vi "MergeTool - Cambridge.vi"(8 "VI Reference":refnum<vi>, 10 "Display References":refnum<vi>[](array[refnum])) -> ()   [LabVIEW 2014]
uses:
  <vilib>/Utility/cursorutil.llb/Set Cursor (Icon Pict).vi
panel:
  in  "Save":bool
  in  "Reset Zoom":bool
  in  "Zoom In":bool
  in  "Pick Blue":bool
  in  "Pick Green":bool
  in  "Pick Red":bool
  in  "Clear All":bool
  out "Merge Image":picture
  in  "Exit":bool
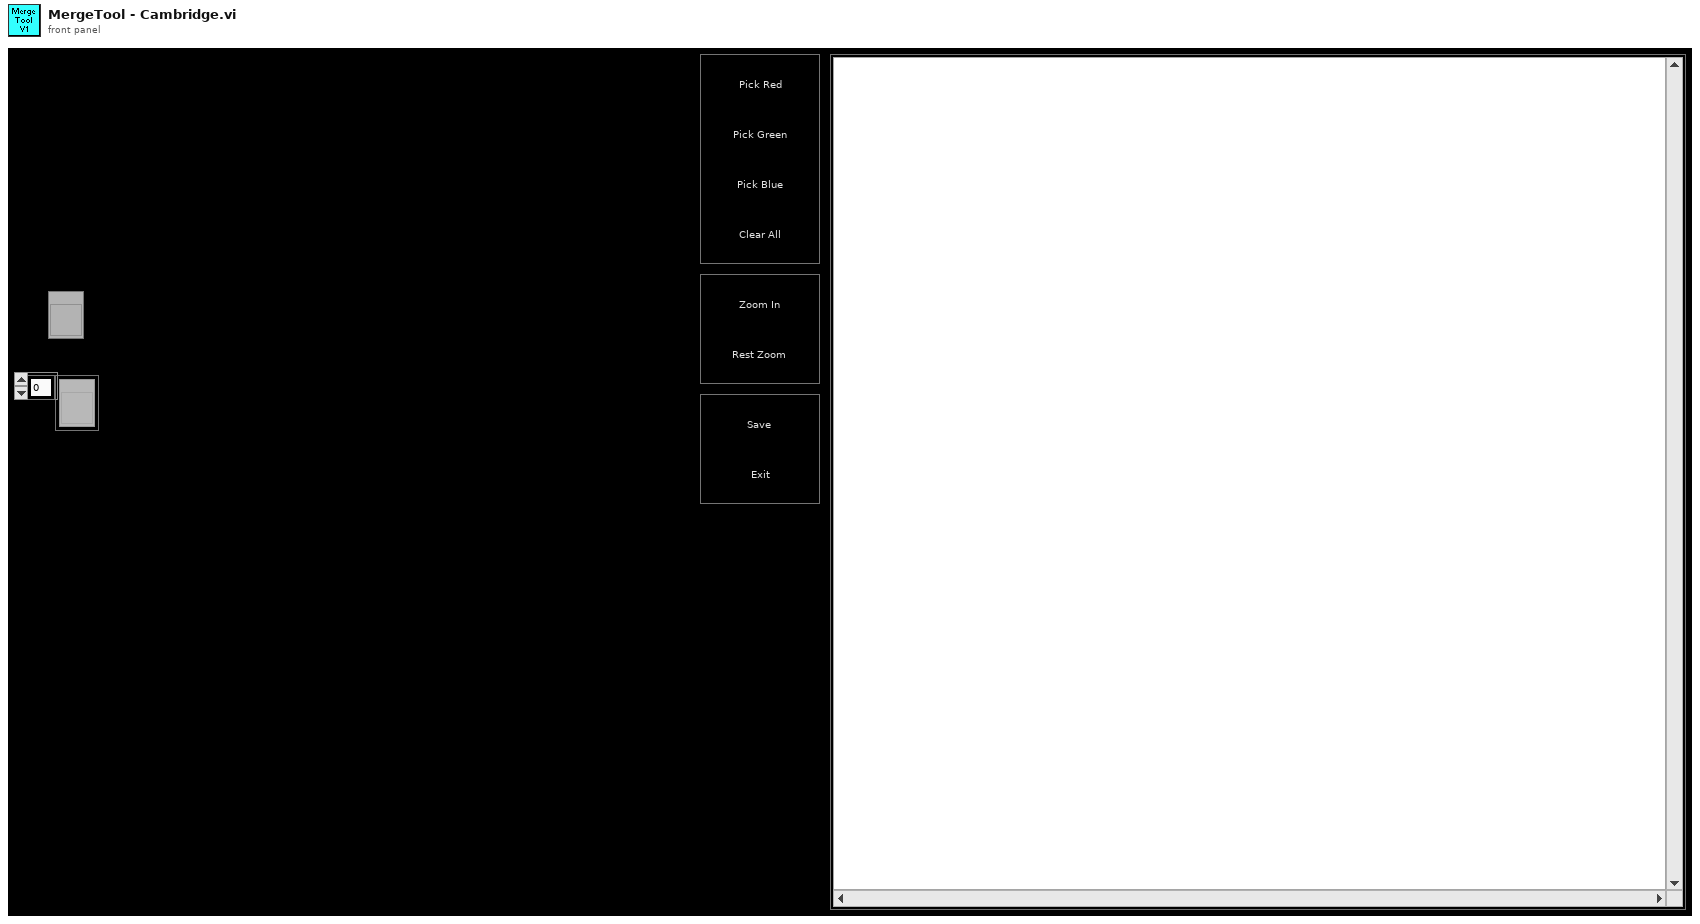
[diagram p1: front panel]
types:
  T1 = typedef "LVBoundsTypeDef.ctl" = cluster{"Width":u32, "Height":u32}
  T2 = typedef "imagedata.ctl" = cluster{"image type":i32, "image depth":i32, "image":u8[], "mask":u8[], "colors":u32[], "Rectangle":cluster{"left":i16, "top":i16, "right":i16, "bottom":i16}}
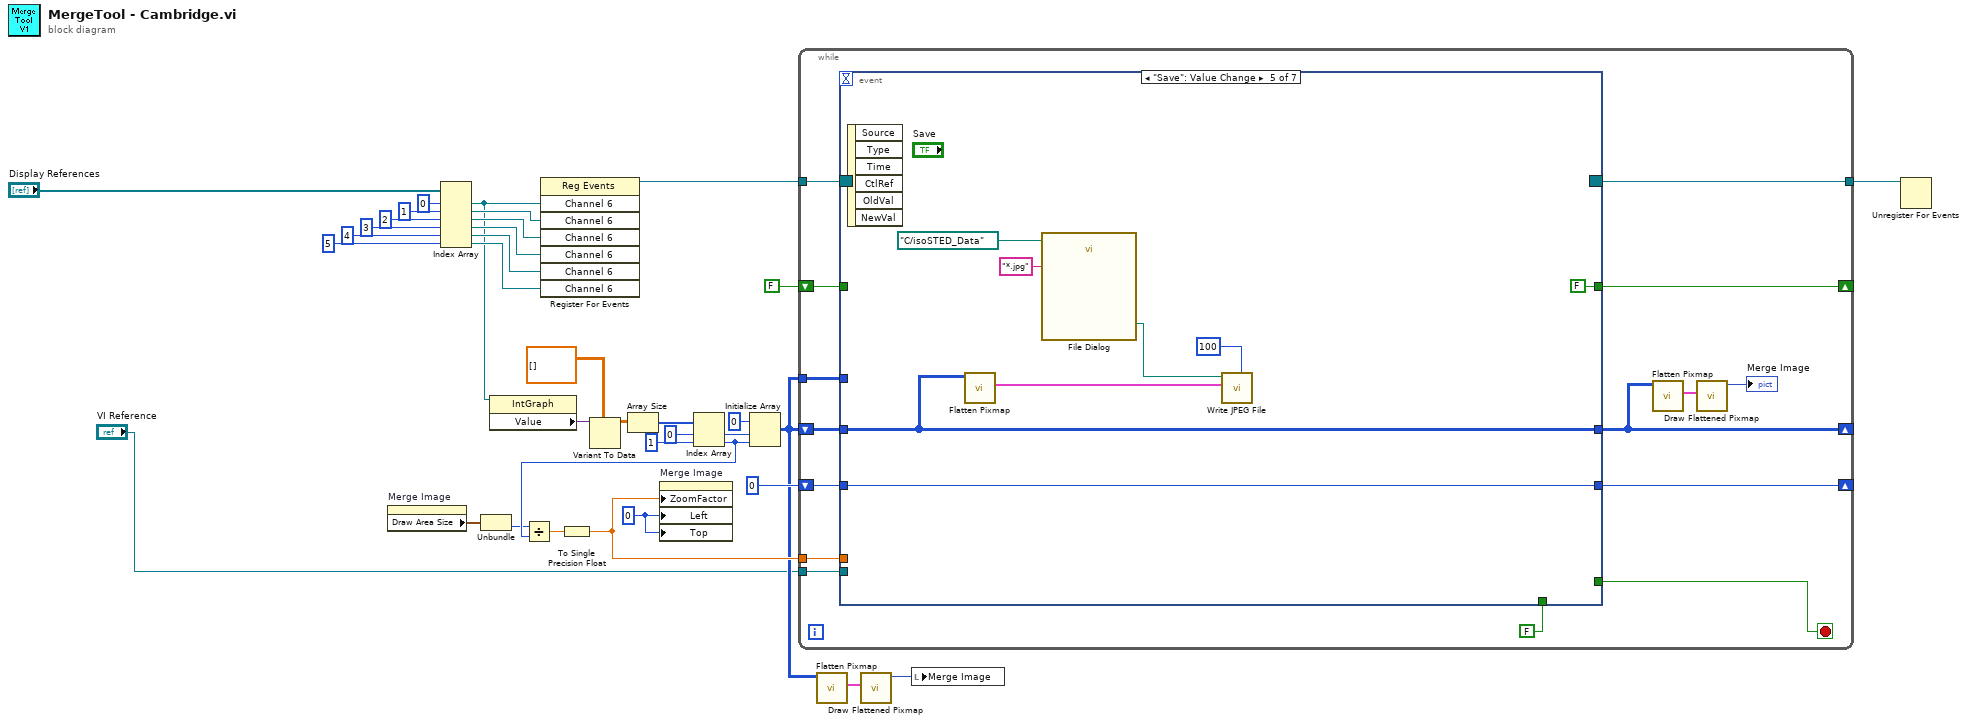
[diagram p0: block diagram]
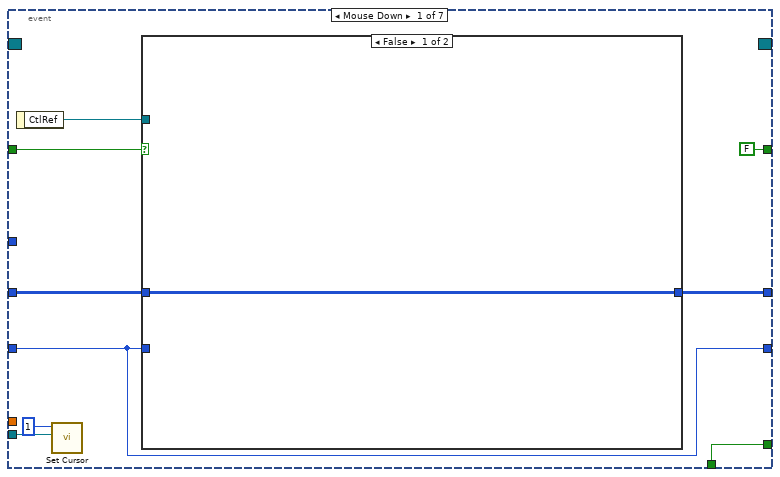
[diagram p2: hidden frame]
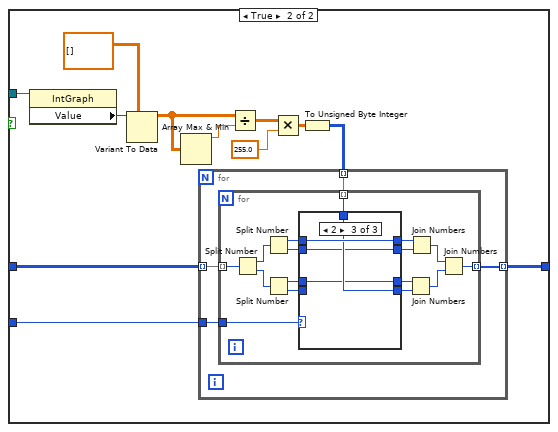
[diagram p3: hidden frame]
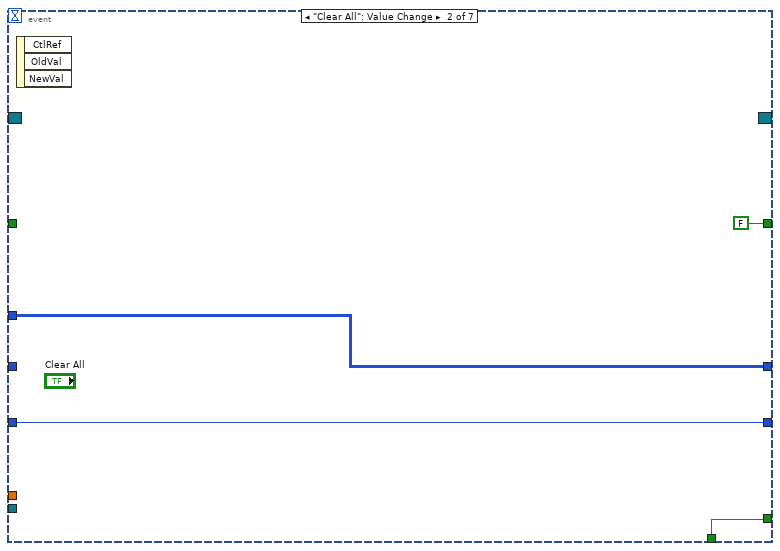
[diagram p6: hidden frame]
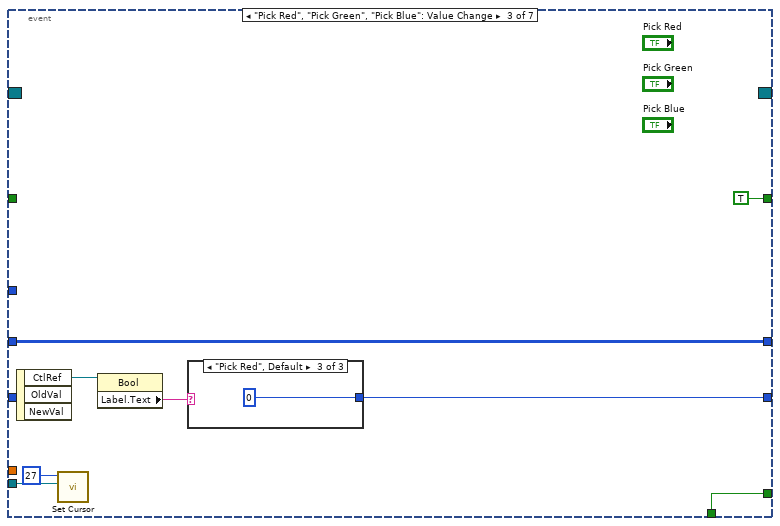
[diagram p7: hidden frame]
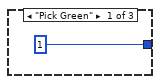
[diagram p8: hidden frame]
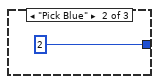
[diagram p9: hidden frame]
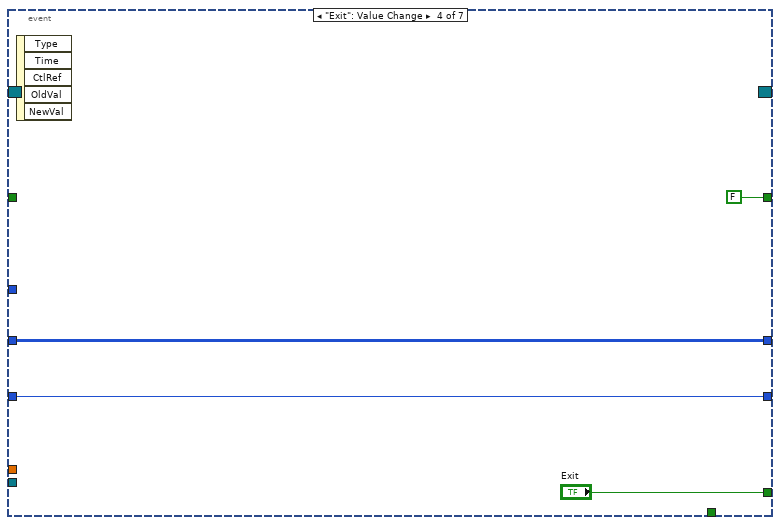
[diagram p10: hidden frame]
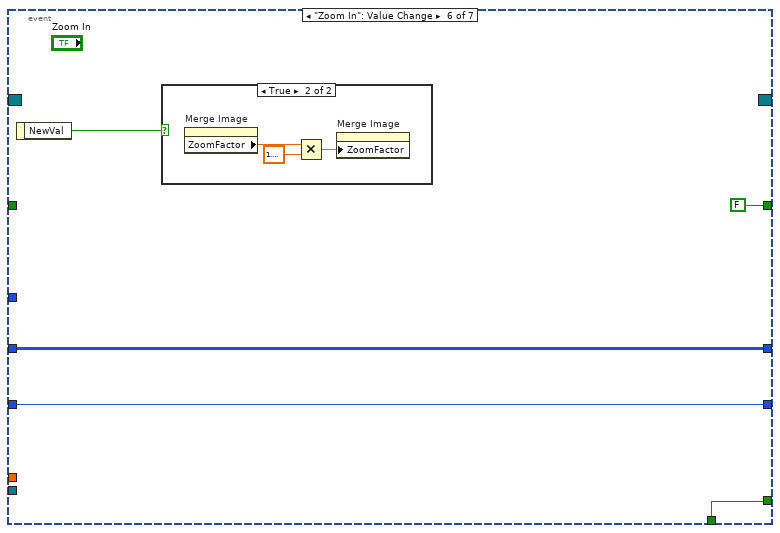
[diagram p11: hidden frame]
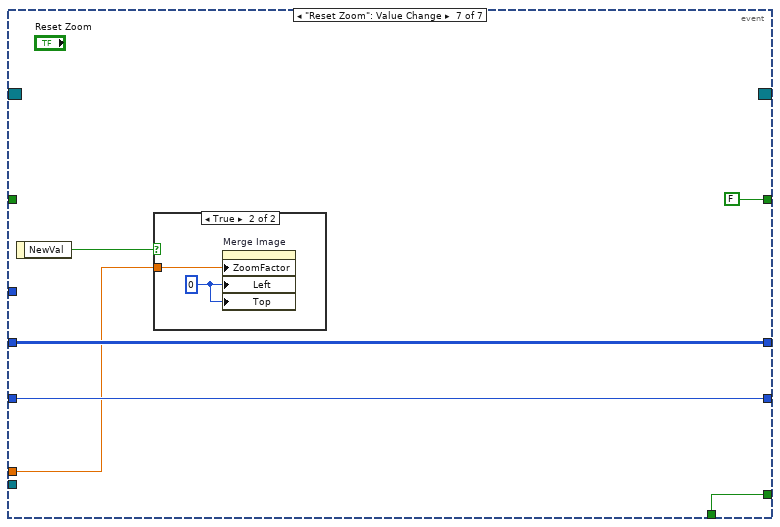
[diagram p13: hidden frame]
diagram:
  w7 = i16 0 ("Origin:Left")
  n1 = property on="Merge Image" class="Pict"() -> ("Draw Area Size"=w12:T1)  [unwired: 2 in, 2 out]
  n2 = Index Array(array="Display References", index #1=0 ("index"), index #2=1 ("index"), index #3=2 ("index"), index #4=3 ("index"), index #5=4 ("index"), index #6=5 ("index")) -> (element #1=w22:refnum<vi>, element #2=w25:refnum<vi>, element #3=w26:refnum<vi>, element #4=w27:refnum<vi>, element #5=w28:refnum<vi>, element #6=w29:refnum<vi>)
  n3 = Unbundle(w12) -> ("Height"=w11:u32)  [unwired: 1 out]
  n4 = property class="IntGraph"(reference=w22) -> ("Value"=w21:variant)  [unwired: 1 in, 2 out]
  n5 = register-events(w22, w25, w26, w27, w28, w29) -> (reference out=w24:refnum<event-registration>)  [unwired: 2 in, 1 out]
  n6 = Variant To Data(type=sgl[][] [], Variant=w21) -> (data=w19:sgl[][])  [unwired: 1 in, 1 out]
  n7 = Array Size(array=w19) -> (size(s)=w18:i32[])
  n8 = Index Array(array=w18, index #1=0 ("index"), index #2=1 ("index")) -> (element #1=w15:i32, element #2=w13:i32)
  n9 = Divide(x=w11, y=w13) -> (x/y=w9:dbl)
  n10 = To Single Precision Float(number=w9) -> (single precision float=w8:sgl)
  n11 = property on="Merge Image" class="Pict"("ZoomFactor"=w8, "Left"=w7, "Top"=w7) -> ()  [unwired: 2 in, 2 out]
  n12 = Initialize Array(u32 0 ("element"), w15, w13) -> (w4:u32[][])
  n13 = while {
    tunnel: w24 -> [w48]
    tunnel: [w47] -> w23
    shift-right: [w42] -> _
    shift-left: w4 -> [w46]
    tunnel: w4 -> [w45]
    tunnel: "VI Reference" -> [w41]
    shift-right: [w40] -> _
    shift-left: u8 0 -> [w39]
    tunnel: w8 -> [w38]
    shift-right: [w37] -> _
    shift-left: FALSE -> [w36]
    stop <- w50 stop-if-true
    n14 = event shown="[4] \"Save\": Value Change" {
      selector: w48 -> [_ _ _ _ _ _ _]
      dyn-events: [_ _ _ _ _ _ _] -> w47
      timeout: _ -> [_ _ _ _ _ _ _]
      tunnel: [w58 w107 w116 "Exit" _ w136 w143] -> w50
      tunnel: FALSE -> [w58 w107 w116 _ _ w136 w143]
      tunnel: w46 -> [w57 _ w115 w122 w129 w134 w145]
      tunnel: [w56 w108 w115 w122 w129 w134 w145] -> w42
      tunnel: w45 -> [_ w108 _ _ _ _ _]
      tunnel: w41 -> [w54 _ w113 _ _ _ _]
      tunnel: [w52 w106 w110 w121 w131 w135 w144] -> w40
      tunnel: w39 -> [w52 w106 _ w121 w131 w135 w144]
      tunnel: w38 -> [_ _ _ _ _ _ w142]
      tunnel: [FALSE FALSE TRUE FALSE FALSE FALSE FALSE] -> w37
      tunnel: w36 -> [w53 _ _ _ _ _ _]
      event Mouse Down {
        n15 = event-data() -> ("CtlRef"=w59:refnum<vi>)  [unwired: 1 in]
        n16 = call-poly <vilib>:"Set Cursor.vi"("VI reference (current VI)"=w54, "icon"=u16 1) -> ()  [unwired: 8 in, 2 out]
        n17 = case shown="False" w53 {
          tunnel: w59 -> [_ w72]
          tunnel: w57 -> [w60 w71]
          tunnel: [w60 w62] -> w56
          tunnel: w52 -> [_ w61]
          frame False {
          }
          frame True {
            n18 = property class="IntGraph"(reference=w72) -> ("Value"=w67:variant)  [unwired: 1 in, 2 out]
            n19 = Variant To Data(type=sgl[][] [], Variant=w67) -> (data=w65:sgl[][])  [unwired: 1 in, 1 out]
            n20 = Array Max & Min(array=w65) -> (max value=w70:sgl)  [unwired: 3 out]
            n21 = Divide(x=w65, y=w70) -> (x/y=w68:sgl[][])
            n22 = Multiply(x=w68, y=sgl 255.0) -> (x*y=w64:sgl[][])
            n23 = To Unsigned Byte Integer(number=w64) -> (unsigned 8bit integer=w63:u8[][])
            n24 = for {
              tunnel: w71 -> [w76] mode=indexing
              tunnel: w63 -> [w75] mode=indexing
              tunnel: [w74] -> w62 mode=indexing
              tunnel: w61 -> [w73]
              n25 = for {
                tunnel: w76 -> [w92] mode=indexing
                tunnel: w75 -> [w81] mode=indexing
                tunnel: [w85] -> w74 mode=indexing
                tunnel: w73 -> [w77]
                n26 = Split Number(x=w92) -> (hi(x)=w91:u16, lo(x)=w90:u16)
                n27 = Split Number(x=w91) -> (hi(x)=w87:u8, lo(x)=w84:u8)
                n28 = Split Number(x=w90) -> (hi(x)=w83:u8, lo(x)=w82:u8)
                n29 = case shown="2" w77 {
                  tunnel: w87 -> [w96 w100 w104]
                  tunnel: [w96 w100 w104] -> w86
                  tunnel: w84 -> [_ w98 w102]
                  tunnel: w83 -> [w94 _ w101]
                  tunnel: w82 -> [w93 w97 _]
                  tunnel: w81 -> [w95 w99 w103]
                  tunnel: [w95 w98 w102] -> w80
                  tunnel: [w94 w99 w101] -> w79
                  tunnel: [w93 w97 w103] -> w78
                  frame 0, Default {
                  }
                  frame 1 {
                  }
                  frame 2 {
                  }
                }
                n30 = Join Numbers(hi=w79, lo=w78) -> ((hi.lo)=w88:u16)
                n31 = Join Numbers(hi=w86, lo=w80) -> ((hi.lo)=w89:u16)
                n32 = Join Numbers(hi=w89, lo=w88) -> ((hi.lo)=w85:u32)
              }
            }
          }
        }
      }
      event "Clear All": Value Change {
        n33 = event-data() -> ()  [unwired: 1 in, 3 out]
      }
      event "Pick Red", "Pick Green", "Pick Blue": Value Change {
        n34 = event-data() -> ("CtlRef"=w112:refnum<vi>)  [unwired: 1 in, 2 out]
        n35 = call-poly <vilib>:"Set Cursor.vi"("VI reference (current VI)"=w113, "icon"=u16 27) -> ()  [unwired: 8 in, 2 out]
        n36 = property class="Bool"(reference=w112) -> ("Label.Text"=w111:string)  [unwired: 1 in, 2 out]
        n37 = case shown="\"Pick Red\", Default" w111 {
          tunnel: [u8 1 u8 2 u8 0] -> w110
          frame "Pick Green" {
          }
          frame "Pick Blue" {
          }
          frame "Pick Red", Default {
          }
        }
      }
      event "Exit": Value Change {
        n38 = event-data() -> ()  [unwired: 1 in, 5 out]
      }
      event "Save": Value Change {
        n39 = event-data() -> ()  [unwired: 1 in, 6 out]
        n40 = call <vilib>:"Flatten Pixmap.vi"("24-bit pixmap"=w129) -> ("image data"=w128:T2)  [unwired: 5 in, 5 out]
        n41 = call "File Dialog"("start path"=path "C:/isoSTED_Data", "pattern (all files)"="*.jpg") -> ("selected path"=w124:path)  [unwired: 10 in, 3 out]
        n42 = call <vilib>:"Write JPEG File.vi"("quality (80)"=100, "image data"=w128, "path to JPEG file"=w124) -> ()  [unwired: 7 in, 2 out]
      }
      event "Zoom In": Value Change {
        n43 = event-data() -> ("NewVal"=w133:bool)  [unwired: 1 in]
        n44 = case shown="True" w133 {
          frame False {
          }
          frame True {
            n45 = property on="Merge Image" class="Pict"() -> ("ZoomFactor"=w139:sgl)  [unwired: 2 in, 2 out]
            n46 = Multiply(x=w139, y=sgl 1.1) -> (x*y=w137:sgl)
            n47 = property on="Merge Image" class="Pict"("ZoomFactor"=w137) -> ()  [unwired: 2 in, 2 out]
          }
        }
      }
      event "Reset Zoom": Value Change {
        n48 = event-data() -> ("NewVal"=w141:bool)  [unwired: 1 in]
        n49 = case shown="True" w141 {
          tunnel: w142 -> [_ w147]
          frame False {
          }
          frame True {
            w146 = i16 0 ("Origin:Left")
            n50 = property on="Merge Image" class="Pict"("ZoomFactor"=w147, "Left"=w146, "Top"=w146) -> ()  [unwired: 2 in, 2 out]
          }
        }
      }
    }
    n51 = call <vilib>:"Flatten Pixmap.vi"("24-bit pixmap"=w42) -> ("image data"=w44:T2)  [unwired: 5 in, 5 out]
    n52 = call <vilib>:"Draw Flattened Pixmap.vi"("image data"=w44) -> ("new picture"=→"Merge Image":picture)  [unwired: 1 in, 7 out]
  }
  n53 = call <vilib>:"Flatten Pixmap.vi"("24-bit pixmap"=w4) -> ("image data"=w6:T2)  [unwired: 5 in, 5 out]
  n54 = call <vilib>:"Draw Flattened Pixmap.vi"("image data"=w6) -> ("new picture"=w5:picture)  [unwired: 1 in, 7 out]
  n55 = local write "Merge Image"(w5) -> ()
  n56 = Unregister For Events(event registration refnum=w23) -> ()  [unwired: 1 in, 1 out]
